vi "Action Queue Consumer.vi"() -> ()   [LabVIEW 2012, in "SlideEngine.lvclass"]
uses:
  SlideEngine.lvclass
  SlideEngine.lvclass/SlideEngine.ctl
panel:
  in  "Control":refnum<vi>
  in  "SlideEngine.lvclass In":refnum<class "SlideEngine.lvclass">
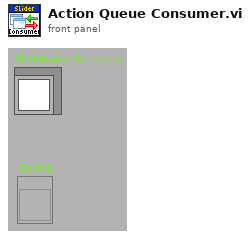
[diagram p1: front panel]
types:
  T1 = typedef "SlideActions.ctl" = enum16{"Left Open", "Left Close"}
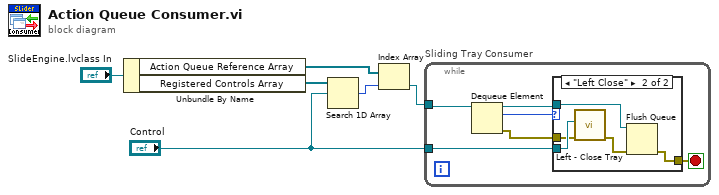
[diagram p0: block diagram]
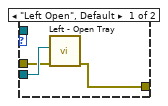
[diagram p2: hidden frame]
diagram:
  n1 = Unbundle By Name("SlideEngine.lvclass In") -> ("Action Queue Reference Array"=w4:refnum<queue>[], "Registered Controls Array"=w5:refnum<vi>[])
  n2 = Search 1D Array(1D array=w5, element="Control") -> (index of element=w3:i32)  [unwired: 1 out]
  n3 = Index Array(array=w4, index=w3) -> (element=w2:refnum<queue>)
  n4 = while "Sliding Tray Consumer" {
    tunnel: w2 -> [w11]
    tunnel: "Control" -> [w9]
    stop <- w12 stop-if-true
    n5 = Dequeue Element(queue=w11) -> (queue out=w10:refnum<queue>, element=w8:T1, error out=w7:errorcluster)  [unwired: 1 in, 2 out]
    n6 = case shown="\"Left Close\"" w8 {
      tunnel: [w15 w16] -> w12
      tunnel: w10 -> [_ w19]
      tunnel: w9 -> [w14 w18]
      tunnel: w7 -> [w13 w17]
      frame "Left Open", Default {
        n7 = call "Left - Open Tray.vi"("error in (no error)"=w13, "Ctl Refnum"=w14) -> ("error out"=w15:errorcluster)  [unwired: 9 out]
      }
      frame "Left Close" {
        n8 = call "Left - Close Tray.vi"("error in (no error)"=w17, "Ctl Refnum"=w18) -> ("error out"=w20:errorcluster)  [unwired: 9 out]
        n9 = Flush Queue(queue=w19, error in (no error)=w20) -> (error out=w16:errorcluster)  [unwired: 2 out]
      }
    }
  }
